vi "OUT.vi"() -> ()   [LabVIEW 2020]
panel:
  in  "out":bool
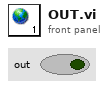
[diagram p1: front panel]
diagram:
